vi "Msg.vi"(7 "Queue Actor in":refnum<class "Queue Actor.lvclass">, 11 "String Indicator Msg in":refnum<class "String Indicator Msg.lvclass">) -> (5 "Queue Actor out":refnum<class "Queue Actor.lvclass">)   [LabVIEW 2021, in "String Indicator Msg.lvlib" / "String Indicator Msg.lvclass"]
uses:
  String Indicator Msg.lvclass
  Actor/Queue Actor/Queue Actor.lvclass
  String Indicator/String Indicator.lvclass
  String Indicator Msg.lvclass/String Indicator Msg.ctl
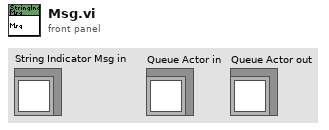
[diagram p1: front panel]
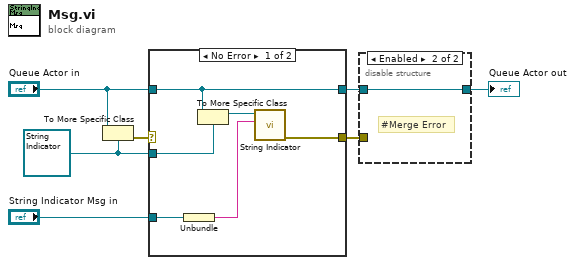
[diagram p0: block diagram]
diagram:
  w6 = refnum<class "String Indicator.lvclass"> refnum ("String Indicator Ref.lvlib:String Indicator.lvclass")
  n1 = To More Specific Class(target class=w6, reference="Queue Actor in") -> (error out=w7:errorcluster)  [unwired: 1 in, 1 out]
  n2 = case shown="No Error" w7 {
    selector: w7 -> [_ w14]
    tunnel: [w10 w15] -> w5
    tunnel: "Queue Actor in" -> [w10 w15]
    tunnel: w6 -> [w13 _]
    tunnel: "String Indicator Msg in" -> [w9 _]
    tunnel: [w11 w14] -> w4
    frame No Error {
      n3 = Unbundle(w9) -> (w8:string)
      n4 = To More Specific Class(target class=w13, reference=w10) -> (specific class reference=w12:refnum<class "String Indicator.lvclass">)  [unwired: 1 in, 1 out]
      n5 = call-dynamic "String Indicator.vi"("String Indicator"=w8, "String Indicator in"=w12) -> ("error out"=w11:errorcluster)  [unwired: 9 in]
    }
    frame Error {
    }
  }
  n6 = disable-structure shown="Enabled" {
    disable-tunnel: [w16 w17] -> w2
    disable-tunnel: w5 -> [w16 w17]
    disable-tunnel: w4 -> [_ _]
    frame Disabled {
    }
    frame Enabled {
      # "#Merge Error"
    }
  }
  "Queue Actor out" <- w2
